vi "OAT Easy Significant Gabor Order Tracking.vi"   [LabVIEW 2017]
doc: "Extracts the most significant orders from <B>scaled signal [EU]</B> and computes <B>magnitudes</B> and <B>phase lags</B> for the significant orders. You can use this polymorphic VI to perform significant order tracking for an analog tachometer signal or a digital tachometer signal. The data type you wire to the <B>analog tach signal</B> input determines the polymorphic instance to use."
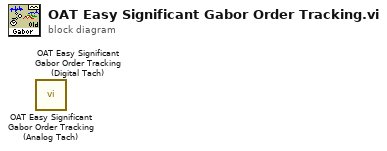
[diagram p0: block diagram]
diagram:
  n1 = call <vilib>:"OAT Easy Significant Gabor Order Tracking (Analog Tach).vi"() -> ()  [unwired: 9 in, 7 out]
  n2 = call <vilib>:"OAT Easy Significant Gabor Order Tracking (Digital Tach).vi"() -> ()  [unwired: 9 in, 7 out]
